vi "rethinkdb_example_simple.vi"() -> ()   [LabVIEW 2017]
uses:
  rethinkdb/msg/rethinkdb_msg_connect_auth.ctl
  rethinkdb/json/json_element.ctl
  rethinkdb/json/json_element_type.ctl
  rethinkdb/json/json_parse_value.vi
panel:
  out "elements":T1[](array[typedef])
  out "error decode":errorcluster
  out "response_json":string
  in  "query":string="[1,\"foo\",{}]"
  in  "query_token":u64=1 format="%016x"
  out "server_signature":string
  in  "auth":T3={"user"="bob", "password"="bob"}
  in  "host (\"localhost\")":string="localhost"
  in  "port (28015)":u16=28015
  in  "ms timeout (10000)":i32=10000
  out "error out":errorcluster
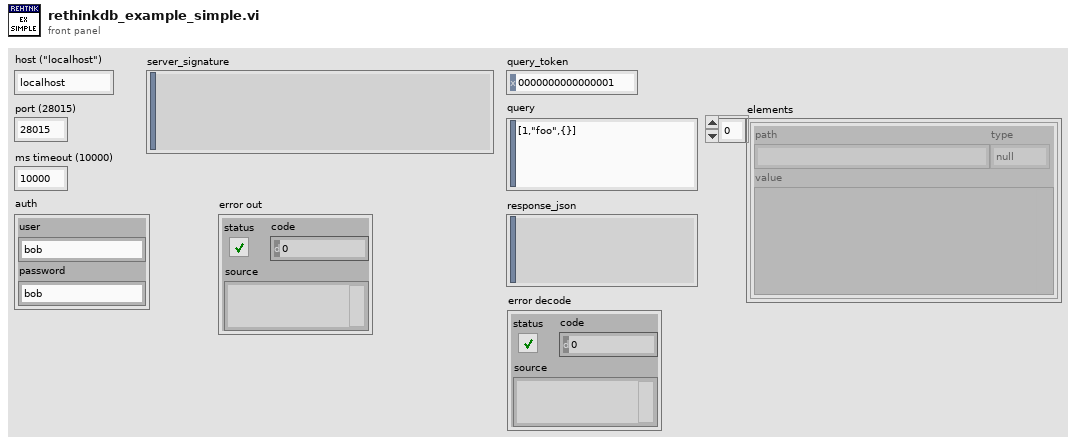
[diagram p1: front panel]
types:
  T1 = typedef "json_element.ctl" = cluster{"path":string, "type":T2, "value":variant}
  T2 = typedef "json_element_type.ctl" = enum8{"null", "bool", "int", "uint", "float", "string", "array", "object"}
  T3 = typedef "rethinkdb_msg_connect_auth.ctl" = cluster{"user":string, "password":string}
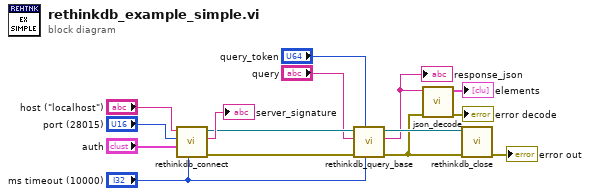
[diagram p0: block diagram]
diagram:
  n1 = call "rethinkdb_connect.vi"("ms timeout (10000)"="ms timeout (10000)", "auth"="auth", "port (28015)"="port (28015)", "host (\"localhost\")"="host (\"localhost\")") -> ("error out"=w10:errorcluster, "server_signature"=→"server_signature":string, "rethinkdb"=w9:refnum<k5>)  [unwired: 5 in]
  n2 = call "rethinkdb_query_base.vi"("timeout ms (10000)"="ms timeout (10000)", "query_token"="query_token", "error in (no error)"=w10, "query"="query", "rethinkdb in"=w9) -> ("error out"=w2:errorcluster, "response_json"=w4:string, "rethinkdb out"=w8:refnum<k5>)  [unwired: 2 in, 2 out]
  "response_json" <- w4
  n3 = call "json_decode.vi"("error in (no error)"=w2, "json"=w4) -> ("error out"=→"error decode":errorcluster, "elements"=→"elements":T1[])  [unwired: 8 in]
  n4 = call "rethinkdb_close.vi"("error in (no error)"=w2, "rethinkdb in"=w8) -> ("error out"=→"error out":errorcluster)  [unwired: 9 in]
